vi "Get Char Index.vi"(8 "error in (no error)":errorcluster, 10 "charcode":u32, 11 "face":i64) -> (0 "error out":errorcluster, 2 "index":u32, 3 "face out":i64)   [LabVIEW 2023, in "Freetype Drawer.lvlib"]
uses:
  Freetype Drawer.lvlib
  libfreetype.dll
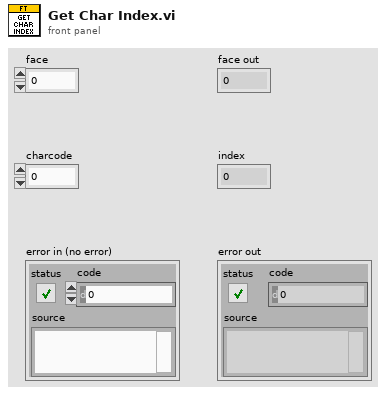
[diagram p1: front panel]
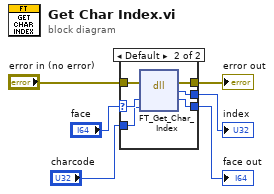
[diagram p0: block diagram]
diagram:
  n1 = case shown="Default" "face" {
    selector: "face" -> [w7 w11]
    tunnel: "error in (no error)" -> [w8 w14]
    tunnel: [_ w13] -> w5
    tunnel: [w8 w12] -> w4
    tunnel: [w7 w10] -> w2
    tunnel: "charcode" -> [_ w9]
    frame 0 {
    }
    frame Default {
      n2 = dll-call lib="E:/Labview/LV 2023/Libs/LV Symbol/Freetype Drawer/libfreetype.dll" fn="FT_Get_Char_Index"(error in=w14, "face"=w11, "charcode"=w9) -> (error out=w12:errorcluster, "index"=w13:u32, "face"=w10:i64)  [unwired: 3 in, 1 out]
    }
  }
  "index" <- w5
  "error out" <- w4
  "face out" <- w2
